vi "Auto_IV_CV_XML_Excell_Label.vi"(9 "Cluster":T1, 10 "Loop Count":i32, 11 "IV or CV":i32) -> (1 "File Name":string, 2 "Excell Cell Title":string[](array[string]), 3 "XML Data Tags":string[](array[string]))   [LabVIEW 2009]
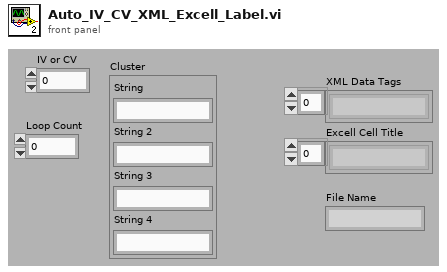
[diagram p1: front panel]
types:
  T1 = cluster{"String":string, "String 2":string, "String 3":string, "String 4":string}
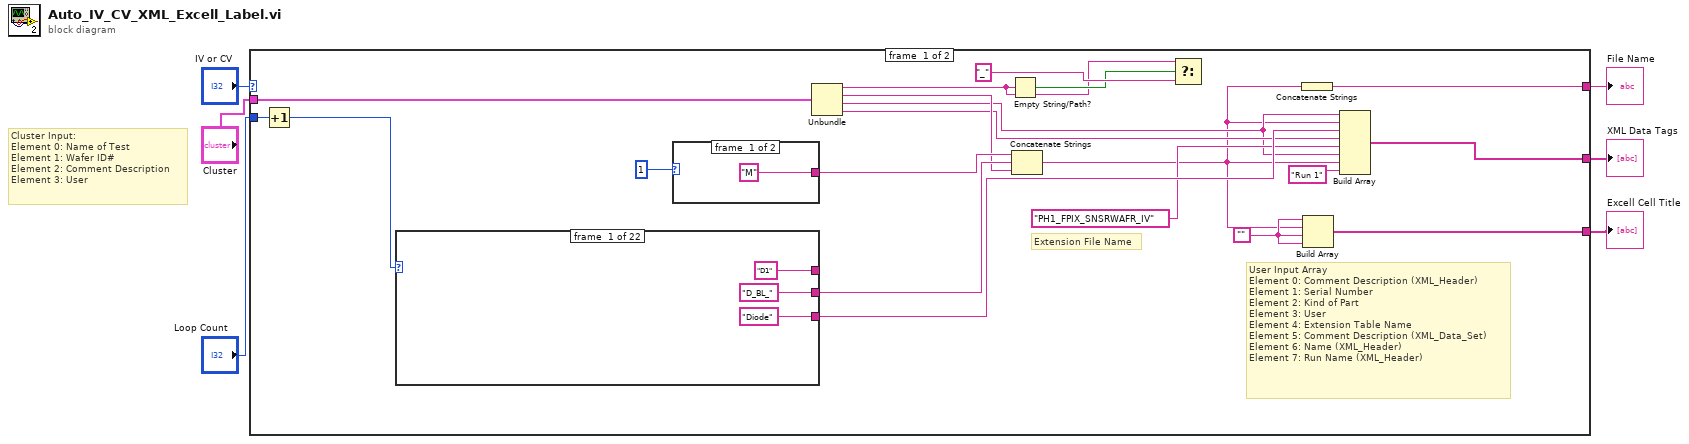
[diagram p0: block diagram]
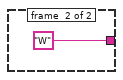
[diagram p2: hidden frame]
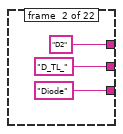
[diagram p3: hidden frame]
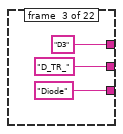
[diagram p4: hidden frame]
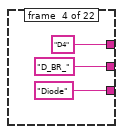
[diagram p5: hidden frame]
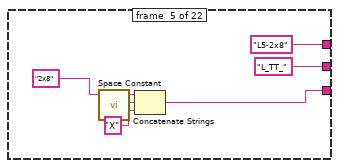
[diagram p6: hidden frame]
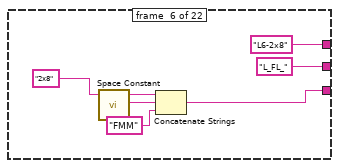
[diagram p7: hidden frame]
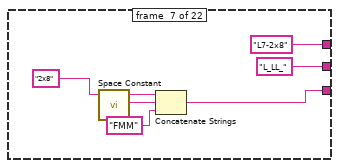
[diagram p8: hidden frame]
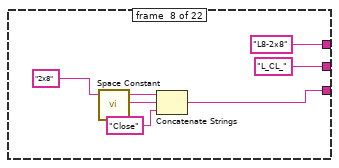
[diagram p9: hidden frame]
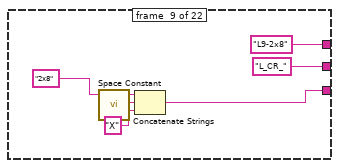
[diagram p10: hidden frame]
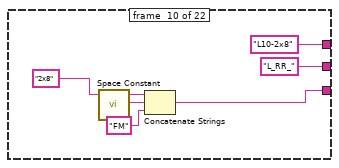
[diagram p11: hidden frame]
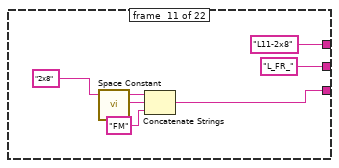
[diagram p12: hidden frame]
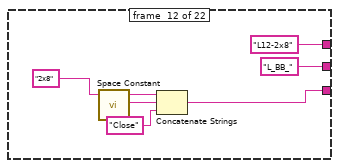
[diagram p13: hidden frame]
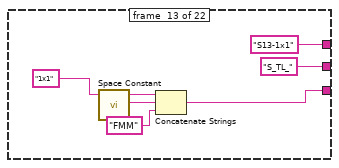
[diagram p14: hidden frame]
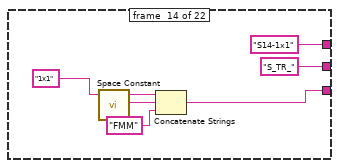
[diagram p15: hidden frame]
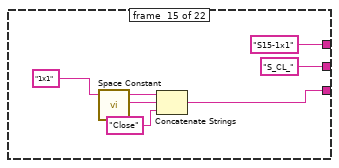
[diagram p16: hidden frame]
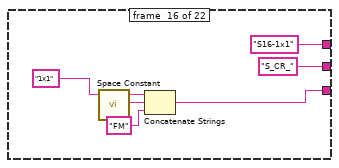
[diagram p17: hidden frame]
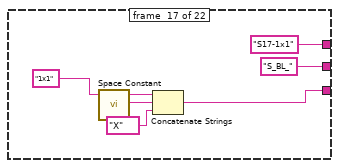
[diagram p18: hidden frame]
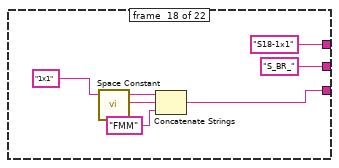
[diagram p19: hidden frame]
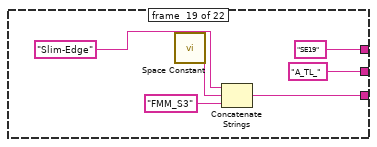
[diagram p20: hidden frame]
diagram:
  # "Cluster Input:\nElement 0: Name of Test\nElement 1: Wafer ID#\nElement 2: Comment Description\nElement 3: User"
  n1 = case shown="0, Default" "IV or CV" {
    tunnel: "Cluster" -> [w18 w153]
    tunnel: [w16 w150] -> w3
    tunnel: [w15 w151] -> w4
    tunnel: [w13 w152] -> w2
    tunnel: "Loop Count" -> [w14 w149]
    frame #0 {
      w22 = ""
      # "Extension File Name"
      # "User Input Array\nElement 0: Comment Description (XML_Header)\nElement 1: Serial Number\nElement 2: Kind of Part\nElement 3: User\nElement 4: Extension Table Name\nElement 5: Comment Description (XML_Data_Set)\nElement 6: Name (XML_Header)\nElement 7: Run Name (XML_Header)"
      n2 = Increment(x=w14) -> (x+1=w26:i32)
      n3 = case shown="5" w26 {
        tunnel: ["D_BL_" "D_TL_" "D_TR_" "D_BR_" "L_TT_" "L_FL_" "L_LL_" "L_CL_" "L_CR_" "L_RR_" "L_FR_" "L_BB_" "S_TL_" "S_TR_" "S_CL_" "S_CR_" "S_BL_" "S_BR_" "A_TL_" "A_TR_" "A_BL_" "A_BR_"] -> w25
        tunnel: ["Diode" "Diode" "Diode" "Diode" w43 w49 w55 w61 w67 w73 w79 w85 w91 w97 w103 w109 w115 w121 w127 w134 w140 w146] -> w12
        tunnel: ["D1" "D2" "D3" "D4" "L5-2x8" "L6-2x8" "L7-2x8" "L8-2x8" "L9-2x8" "L10-2x8" "L11-2x8" "L12-2x8" "S13-1x1" "S14-1x1" "S15-1x1" "S16-1x1" "S17-1x1" "S18-1x1" "SE19" "SE20" "SE21" "SE22"] -> _
        frame #0 {
        }
        frame #1 {
        }
        frame #2 {
        }
        frame #3 {
        }
        frame #4 {
          n4 = call <vilib>:"Space Constant.vi"() -> ("String"=w45:string)
          n5 = Concatenate Strings("2x8", w45, "X") -> (w43:string)
        }
        frame #5 {
          n6 = call <vilib>:"Space Constant.vi"() -> ("String"=w51:string)
          n7 = Concatenate Strings("2x8", w51, "FMM") -> (w49:string)
        }
        frame #6 {
          n8 = call <vilib>:"Space Constant.vi"() -> ("String"=w57:string)
          n9 = Concatenate Strings("2x8", w57, "FMM") -> (w55:string)
        }
        frame #7 {
          n10 = call <vilib>:"Space Constant.vi"() -> ("String"=w63:string)
          n11 = Concatenate Strings("2x8", w63, "Close") -> (w61:string)
        }
        frame #8 {
          n12 = call <vilib>:"Space Constant.vi"() -> ("String"=w69:string)
          n13 = Concatenate Strings("2x8", w69, "X") -> (w67:string)
        }
        frame #9 {
          n14 = call <vilib>:"Space Constant.vi"() -> ("String"=w75:string)
          n15 = Concatenate Strings("2x8", w75, "FM") -> (w73:string)
        }
        frame #10 {
          n16 = call <vilib>:"Space Constant.vi"() -> ("String"=w81:string)
          n17 = Concatenate Strings("2x8", w81, "FM") -> (w79:string)
        }
        frame #11 {
          n18 = call <vilib>:"Space Constant.vi"() -> ("String"=w87:string)
          n19 = Concatenate Strings("2x8", w87, "Close") -> (w85:string)
        }
        frame #12 {
          n20 = call <vilib>:"Space Constant.vi"() -> ("String"=w93:string)
          n21 = Concatenate Strings("1x1", w93, "FMM") -> (w91:string)
        }
        frame #13 {
          n22 = call <vilib>:"Space Constant.vi"() -> ("String"=w99:string)
          n23 = Concatenate Strings("1x1", w99, "FMM") -> (w97:string)
        }
        frame #14 {
          n24 = call <vilib>:"Space Constant.vi"() -> ("String"=w105:string)
          n25 = Concatenate Strings("1x1", w105, "Close") -> (w103:string)
        }
        frame #15 {
          n26 = call <vilib>:"Space Constant.vi"() -> ("String"=w111:string)
          n27 = Concatenate Strings("1x1", w111, "FM") -> (w109:string)
        }
        frame #16 {
          n28 = call <vilib>:"Space Constant.vi"() -> ("String"=w117:string)
          n29 = Concatenate Strings("1x1", w117, "X") -> (w115:string)
        }
        frame #17 {
          n30 = call <vilib>:"Space Constant.vi"() -> ("String"=w123:string)
          n31 = Concatenate Strings("1x1", w123, "FMM") -> (w121:string)
        }
        frame #18 {
          n32 = call <vilib>:"Space Constant.vi"() -> ("String"=w129:string)
          n33 = Concatenate Strings("Slim-Edge", w129, "FMM_S3") -> (w127:string)
        }
        frame #19 {
          n34 = call <vilib>:"Space Constant.vi"() -> ("String"=w135:string)
          n35 = Concatenate Strings("Slim-Edge", w135, "FMM_S3") -> (w134:string)
        }
        frame #20 {
          n36 = call <vilib>:"Space Constant.vi"() -> ("String"=w141:string)
          n37 = Concatenate Strings("Slim-Edge", w141, "FMM_S3") -> (w140:string)
        }
        frame #21 {
          n38 = call <vilib>:"Space Constant.vi"() -> ("String"=w147:string)
          n39 = Concatenate Strings("Slim-Edge", w147, "FMM_S3") -> (w146:string)
        }
      }
      n40 = case shown="1, Default" u16 1 ("Ring") {
        tunnel: ["M" "W"] -> w20
        frame #0 {
        }
        frame #1 {
        }
      }
      n41 = Unbundle(w18) -> ("String"=w21:string, "String 2"=w19:string, "String 3"=w9:string, "String 4"=w11:string)
      n42 = Empty String/Path?(string/path=w21) -> (empty?=w23:bool)
      n43 = Concatenate Strings(w20, w25, w19) -> (w7:string)
      n44 = Select(t=w21, s=w23, f="_" ("string")) -> ()  [unwired: 1 out]
      n45 = Concatenate Strings(w7) -> (w13:string)
      n46 = Build Array(w22, w7, w22, w22) -> (w16:string[])
      n47 = Build Array(w9, w7, w12, w11, "PH1_FPIX_SNSRWAFR_IV", w9, w7, "Run 1" ("element")) -> (w15:string[])
    }
    frame #1 {
      w164 = ""
      # "Extension File Name"
      # "User Input Array\nElement 0: Comment Description (XML_Header)\nElement 1: Serial Number\nElement 2: Kind of Part\nElement 3: User\nElement 4: Extension Table Name\nElement 5: Comment Description (XML_Data_Set)\nElement 6: Name (XML_Header)\nElement 7: Run Name (XML_Header)"
      n48 = Increment(x=w149) -> (x+1=w168:i32)
      n49 = case shown="6" w168 {
        tunnel: ["D_BL_" "D_TL_" "D_TR_" "D_BR_" "L_TT_" "L_FL_" "L_LL_" "L_CL_" "L_CR_" "L_RR_" "L_FR_" "L_BB_" "S_TL_" "S_TR_" "S_CL_" "S_CR_" "S_BL_" "S_BR_" "A_TL_" "A_TR_" "A_BL_" "A_BR_"] -> w167
        tunnel: ["Diode" "Diode" "Diode" "Diode" w185 w191 w197 w203 w209 w215 w221 w227 w233 w239 w245 w251 w257 w263 w269 w276 w282 w288] -> w159
        tunnel: ["D1" "D2" "D3" "D4" "L5-2x8" "L6-2x8" "L7-2x8" "L8-2x8" "L9-2x8" "L10-2x8" "L11-2x8" "L12-2x8" "S13-1x1" "S14-1x1" "S15-1x1" "S16-1x1" "S17-1x1" "S18-1x1" "SE19" "SE20" "SE21" "SE22"] -> _
        frame #0 {
        }
        frame #1 {
        }
        frame #2 {
        }
        frame #3 {
        }
        frame #4 {
          n50 = call <vilib>:"Space Constant.vi"() -> ("String"=w187:string)
          n51 = Concatenate Strings("2x8", w187, "X") -> (w185:string)
        }
        frame #5 {
          n52 = call <vilib>:"Space Constant.vi"() -> ("String"=w193:string)
          n53 = Concatenate Strings("2x8", w193, "FMM") -> (w191:string)
        }
        frame #6 {
          n54 = call <vilib>:"Space Constant.vi"() -> ("String"=w199:string)
          n55 = Concatenate Strings("2x8", w199, "FMM") -> (w197:string)
        }
        frame #7 {
          n56 = call <vilib>:"Space Constant.vi"() -> ("String"=w205:string)
          n57 = Concatenate Strings("2x8", w205, "Close") -> (w203:string)
        }
        frame #8 {
          n58 = call <vilib>:"Space Constant.vi"() -> ("String"=w211:string)
          n59 = Concatenate Strings("2x8", w211, "X") -> (w209:string)
        }
        frame #9 {
          n60 = call <vilib>:"Space Constant.vi"() -> ("String"=w217:string)
          n61 = Concatenate Strings("2x8", w217, "FM") -> (w215:string)
        }
        frame #10 {
          n62 = call <vilib>:"Space Constant.vi"() -> ("String"=w223:string)
          n63 = Concatenate Strings("2x8", w223, "FM") -> (w221:string)
        }
        frame #11 {
          n64 = call <vilib>:"Space Constant.vi"() -> ("String"=w229:string)
          n65 = Concatenate Strings("2x8", w229, "Close") -> (w227:string)
        }
        frame #12 {
          n66 = call <vilib>:"Space Constant.vi"() -> ("String"=w235:string)
          n67 = Concatenate Strings("1x1", w235, "FMM") -> (w233:string)
        }
        frame #13 {
          n68 = call <vilib>:"Space Constant.vi"() -> ("String"=w241:string)
          n69 = Concatenate Strings("1x1", w241, "FMM") -> (w239:string)
        }
        frame #14 {
          n70 = call <vilib>:"Space Constant.vi"() -> ("String"=w247:string)
          n71 = Concatenate Strings("1x1", w247, "Close") -> (w245:string)
        }
        frame #15 {
          n72 = call <vilib>:"Space Constant.vi"() -> ("String"=w253:string)
          n73 = Concatenate Strings("1x1", w253, "FM") -> (w251:string)
        }
        frame #16 {
          n74 = call <vilib>:"Space Constant.vi"() -> ("String"=w259:string)
          n75 = Concatenate Strings("1x1", w259, "X") -> (w257:string)
        }
        frame #17 {
          n76 = call <vilib>:"Space Constant.vi"() -> ("String"=w265:string)
          n77 = Concatenate Strings("1x1", w265, "FMM") -> (w263:string)
        }
        frame #18 {
          n78 = call <vilib>:"Space Constant.vi"() -> ("String"=w271:string)
          n79 = Concatenate Strings("Slim-Edge", w271, "FMM_S3") -> (w269:string)
        }
        frame #19 {
          n80 = call <vilib>:"Space Constant.vi"() -> ("String"=w277:string)
          n81 = Concatenate Strings("Slim-Edge", w277, "FMM_S3") -> (w276:string)
        }
        frame #20 {
          n82 = call <vilib>:"Space Constant.vi"() -> ("String"=w283:string)
          n83 = Concatenate Strings("Slim-Edge", w283, "FMM_S3") -> (w282:string)
        }
        frame #21 {
          n84 = call <vilib>:"Space Constant.vi"() -> ("String"=w289:string)
          n85 = Concatenate Strings("Slim-Edge", w289, "FMM_S3") -> (w288:string)
        }
      }
      n86 = case shown="1, Default" u16 1 ("Ring") {
        tunnel: ["M" "W"] -> w162
        frame #0 {
        }
        frame #1 {
        }
      }
      n87 = Unbundle(w153) -> ("String"=w163:string, "String 2"=w161:string, "String 3"=w156:string, "String 4"=w158:string)
      n88 = Empty String/Path?(string/path=w163) -> (empty?=w165:bool)
      n89 = Concatenate Strings(w162, w167, w161) -> (w154:string)
      n90 = Select(t=w163, s=w165, f="_" ("string")) -> ()  [unwired: 1 out]
      n91 = Concatenate Strings(w154) -> (w152:string)
      n92 = Build Array(w164, w154, w164, w164) -> (w150:string[])
      n93 = Build Array(w156, w154, w159, w158, "PH1_FPIX_SNSRWAFR_CAP", w156, w154, "Run 1" ("element")) -> (w151:string[])
    }
  }
  "XML Data Tags" <- w4
  "Excell Cell Title" <- w3
  "File Name" <- w2
